vi "Verify with Regex Scrubber Count Unique not found.vi"(8 "error in":errorcluster) -> (0 "error out":errorcluster)   [LabVIEW 2020, in "Scrubber.Tests.lvclass"]
uses:
  Scrubber.Tests.lvclass
  Source/Approval Tests/Regex Scrubber Count Unique/Regex Scrubber Count Unique.lvclass
  C:/Users/SAS/Desktop/ApprovalTests.LabVIEW/Source/Approval Tests/Scrubber/Scrubber.lvclass
  Source/Approval Tests/Options/Options.lvclass
  Source/Approval Tests/Regex Scrubber Count Unique/Regex Scrubber Count Unique.lvclass/Regex Scrubber Count Unique.ctl
  Source/Approval Tests/Options/Options.lvclass/Options.ctl
  Source/Approval Tests/Naming Data/Naming Data.lvclass/Naming Data.ctl
  4b862e9e-fcb2-487f-ab73-d9f83fbf4d2c.vi
  Source/Approval Tests/Regex Scrubber Count Unique/Write Regex.vi
  Source/Approval Tests/Regex Scrubber Count Unique/Write Prefix.vi
  4b862e9e-fcb2-487f-ab73-d9f83fbf4d2c.vi/500b534b-d6f0-4fa5-90b2-c40158375321.vi
  Source/Approval Tests/Update Test Name if Not Defined.vi
  4b862e9e-fcb2-487f-ab73-d9f83fbf4d2c.vi/500b534b-d6f0-4fa5-90b2-c40158375321.vi/93c5622b-9fb7-41e0-8c76-3fde37e94e34.vi
  Source/Approval Tests/Verify Core.vi
  Source/Approval Tests/Options/Read Scrubber.vi
  Source/Approval Tests/Naming Data/Read Test VI Name.vi
  Source/Approval Tests/Naming Data/Write Test VI Name.vi
  Source/Approval Tests/Options/Read Namer.vi
  Source/Approval Tests/Options/Read Naming Data.vi
  Source/Approval Tests/Options/Read Reporter.vi
  Source/Approval Tests/Options/Write Add Scrubber.vi
  Source/Approval Tests/conv EOL.vi
  <vilib>/Utility/libraryn.llb/Check if File or Folder Exists.vi
  Source/Approval Tests/Reporter/Report.vi
  <vilib>/addons/_JKI Toolkits/Caraya/classes/Assert/Assert.vi
  <vilib>/addons/_JKI Toolkits/Caraya/classes/Assert/Assert True.vi
  Source/Approval Tests/Scrubber/Scrubber.lvclass
  Source/Approval Tests/Namer/Namer.lvclass
  Source/Approval Tests/Naming Data/Naming Data.lvclass
  Source/Approval Tests/Reporter/Reporter.lvclass
  Scrubber.Tests.lvclass/Scrubber.Tests.ctl
  <vilib>/addons/_JKI Toolkits/Caraya/classes/Test/Test.lvclass
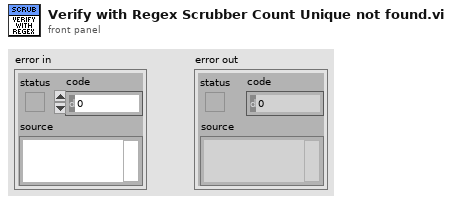
[diagram p1: front panel]
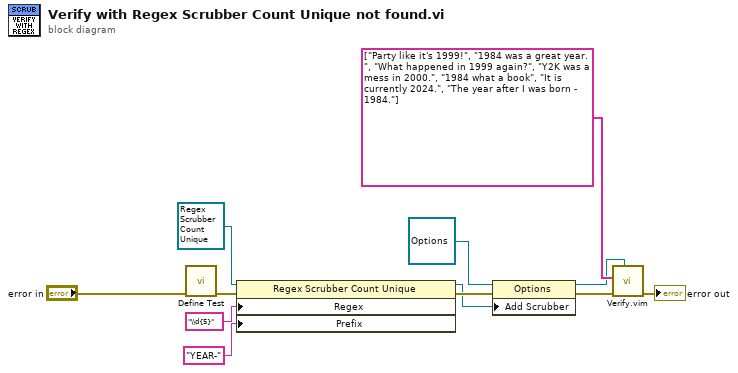
[diagram p0: block diagram]
diagram:
  n1 = call <vilib>:"Define Test.vi"("error in (no error)"="error in") -> ("error out"=w12:errorcluster)  [unwired: 9 in, 1 out]
  n2 = property on="Property Node" class="Regex Scrubber Count Unique"(reference=refnum<class "Regex Scrubber Count Unique.lvclass"> refnum ("Approval Tests.lvlib:Regex Scrubber with Numbered Replacement.lvclass"), error in=w12, "Regex"="\\d{5}", "Prefix"="YEAR-" ("Replacement")) -> (reference out=w2:refnum<class "Regex Scrubber Count Unique.lvclass">, error out=w9:errorcluster)
  n3 = property class="Options"(reference=refnum<class "Options.lvclass"> refnum ("Approval Tests.lvlib:Options.lvclass"), error in=w9, "Add Scrubber"=w2) -> (reference out=w1:refnum<class "Options.lvclass">, error out=w8:errorcluster)
  n4 = call "Verify.vim"("Options"=w1, "error in"=w8, "Test Data"=string[] ["Party like it's 1999!", "1984 was a great year.", "What happened in 1999 again?", "Y2K was a mess in 2000.", "1984 what a book", "It is currently 2024.", "The year after I was born - 1984."]) -> ("error out"=→"error out":errorcluster)  [unwired: 7 in, 1 out]
